vi "Modes and States.vi"(11 "Robot Controls":T5) -> (0 "Step Deployment SS State":T1, 2 "Stacking SS State":T3, 3 "Drive SS State":T4, 5 "Robot Mode":T2)   [LabVIEW 2014]
uses:
  Robot Commands.ctl
  Drive SS/Drive SS State.ctl
  Stacking SS/Stacking SS State.ctl
  Robot Mode.ctl
  Step Deployment SS/Step Deployment SS State.ctl
panel:
  # "Field Centric"
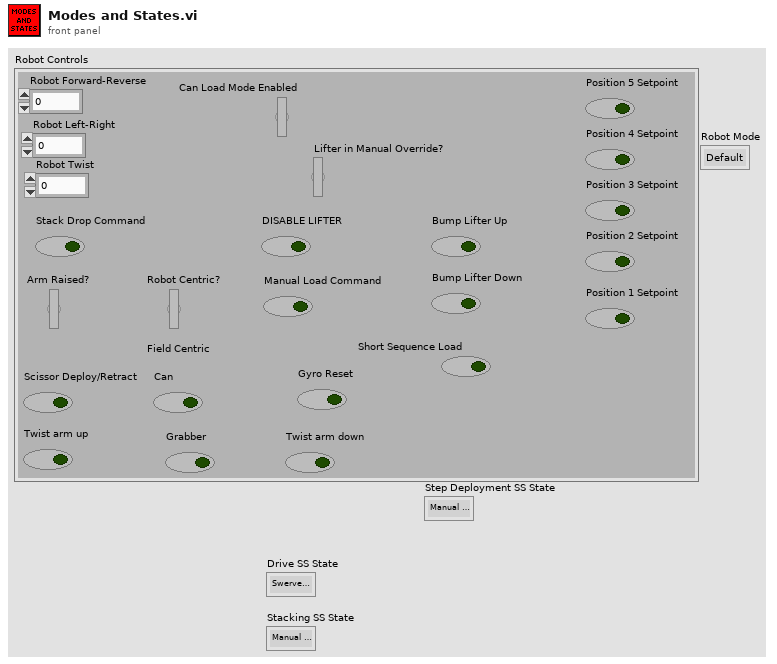
[diagram p1: front panel]
types:
  T1 = typedef "Step Deployment SS State.ctl" = enum16{"Manual Override", "Disabled"}
  T2 = typedef "Robot Mode.ctl" = enum16{"Default", "Manual Override"}
  T3 = typedef "Stacking SS State.ctl" = enum16{"Manual Load", "Manual Override"}
  T4 = typedef "Drive SS State.ctl" = enum16{"Swerve Drive", "Arcade Drive", "Mecanum Drive"}
  T5 = typedef "Robot Commands.ctl" = cluster{"Robot Forward-Reverse":dbl, "Robot Left-Right":dbl, "Robot Twist":dbl, "Can Load Mode Enabled":bool, "Lifter in Manual Override?":bool, "Stack Drop Command":bool, "Arm Raised?":bool, "DISABLE LIFTER":bool, "Position 1 Setpoint":bool, "Position 2 Setpoint":bool, "Position 3 Setpoint":bool, "Position 4 Setpoint":bool, "Position 5 Setpoint":bool, "Bump Lifter Down":bool, "Bump Lifter Up":bool, "Manual Load Command":bool, "Robot Centric?":bool, "Scissor Deploy/Retract":bool, "Grabber":bool, "Can":bool, "Twist arm up":bool, "Gyro Reset":bool, "Twist arm down":bool, "Short Sequence Load":bool}
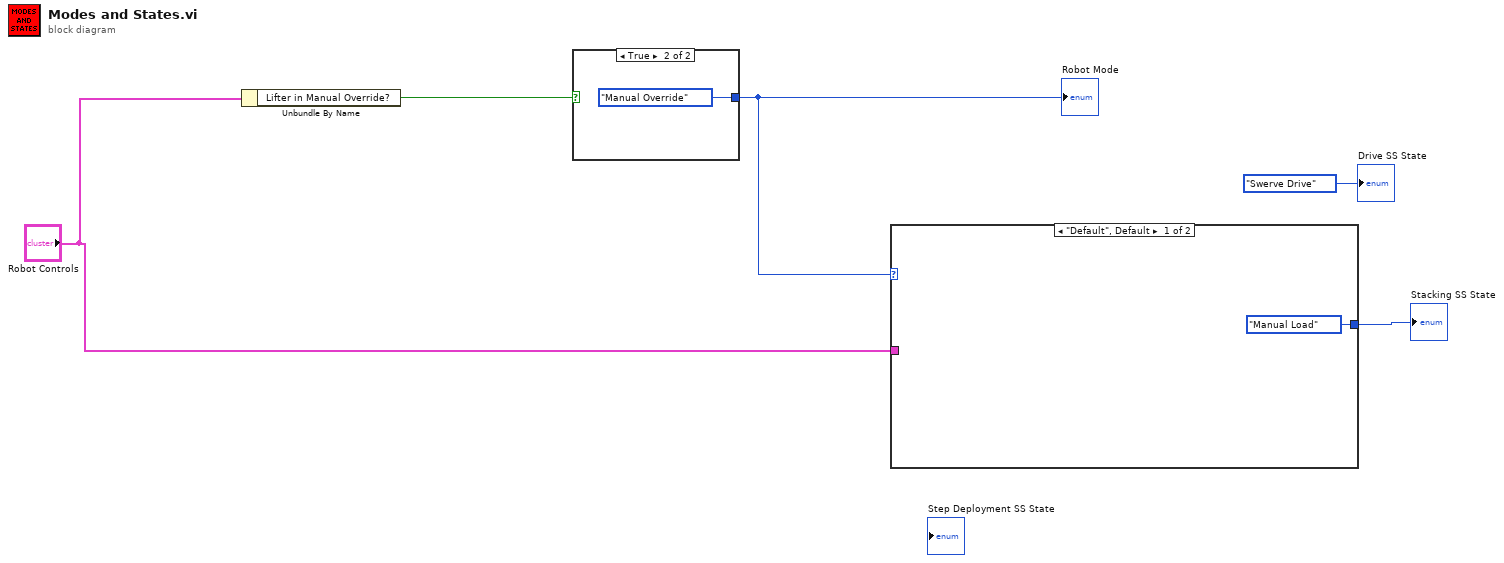
[diagram p0: block diagram]
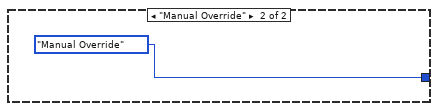
[diagram p2: hidden frame]
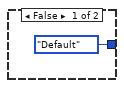
[diagram p3: hidden frame]
diagram:
  n1 = Unbundle By Name("Robot Controls") -> ("Lifter in Manual Override?"=w5:bool)
  n2 = case shown="True" w5 {
    tunnel: [Robot_Mode."Default" ("Robot Mode") Robot_Mode."Manual Override" ("Robot Mode")] -> w1
    frame False {
    }
    frame True {
    }
  }
  "Robot Mode" <- w1
  n3 = case shown="\"Default\", Default" w1 {
    tunnel: [Stacking_SS_State."Manual Load" ("Stacking SS State") Stacking_SS_State."Manual Override" ("Stacking SS State")] -> w3
    tunnel: "Robot Controls" -> [_ _]
    frame "Default", Default {
    }
    frame "Manual Override" {
    }
  }
  "Stacking SS State" <- w3
  "Drive SS State" <- Drive_SS_State."Swerve Drive" ("Drive SS State")
